vi "PH_PPPA_PowerUnit.PC PU on.vi"(0 "i ref in":refnum<vi>, 2 "PU on":bool, 5 "error in (no error)":errorcluster) -> (14 "i ref out":refnum<vi>, 19 "error out":errorcluster)   [LabVIEW 2014, in "PH_PPPA_PowerUnit.lvlib"]
doc: "This is the action VI of the PU on event case. Depending on the inout it does the following:\n\nfalse: set save state\ntrue: if the PreAmp is not disabled and State SM = \"Stand by\", a state change request is send to SM to get \"Switch PU on\" and the attribute \"PU in use\" is set to true. \nelse: GUI Knob is resetted"
uses:
  PH_PPPA_PowerUnit.lvlib
  PH_Basics/PH_PowerUnit_BaseClass/PH_PowerUnit_BaseClass.SM States.ctl
  PH_Basics/PH_PowerUnit_BaseClass/PH_PowerUnit_BaseClass.lvlib
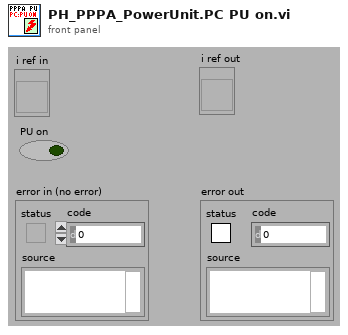
[diagram p1: front panel]
types:
  T1 = typedef "PH_PowerUnit_BaseClass.lvlib/PH_PowerUnit_BaseClass.SM States.ctl" = enum16{".", "Stand by", "Switch PU on", "Configure", "Set Default Voltage", "Set STANDBY", "Set READY", "Wait for Shot Cmd", "Open Dump Rods", "Open Ross Relais", "Close Ross Relais", "Switch PSU on", "Switch PSU off", "Charge", "Switch GD Channel on", "Close Dump Rods", "Rods-TO", "RR-TO", "PSU-TO", "Trigger-TO"}
  T2 = typedef "PH_PPPA_PowerUnit.lvlib/PH_PPPA_PowerUnit.i attribute.ctl" = cluster{"GUI Refs":cluster{"Ignitron":refnum<vi>, "Rossrelais":refnum<vi>, "Set Voltage":refnum<vi>, "PSU":refnum<vi>, "EOC":refnum<vi>, "Trigger":refnum<vi>}, "Ignitron":T3, "PSU":T5, "Dump Ross Relais":T6, "Trigger":cluster{"State Device":T4, "linked?":bool}, "Timing Settings":cluster{"Prdc Fast?":bool, "Default Value Periodic Interval":i32, "Mercury on since":dbl, "Warm up Time Mercury [s]":dbl}, "Set Voltage [V]":dbl, "19er Ignitionbox":string}
  T3 = typedef "PH_PP_Common.lvlib/PH_PP_Common.Ignitron Attributes.ctl" = cluster{"State Device":T4, "linked?":bool}
  T4 = typedef "PH_StatusHandler.lvlib/PH_StatusHandler.Status.ctl" = i16
  T5 = typedef "PH_PP_Common.lvlib/PH_PP_Common.PSU Attributes.ctl" = cluster{"lower limit [V]":dbl, "upper limit [V]":dbl, "Voltage set":bool, "State Device":T4, "linked?":bool}
  T6 = typedef "PH_PP_Common.lvlib/PH_PP_Common.Ross Relais Attributes.ctl" = cluster{"State Device":T4, "linked?":bool}
  T7 = typedef "PH_PowerUnit_BaseClass.lvlib/PH_PowerUnit_BaseClass.i attribute.ctl" = cluster{"Constructor finished":bool, "PU":cluster{"In use":bool, "Service ID in use":i32, "GUI Ref":refnum<vi>}, "Enabling":cluster{"State":T8, "GUI Ref":refnum<vi>}, "Timing":cluster{"Last Shot":dbl, "Time between Shots [Sec]":dbl, "Waiting Time over?":bool, "Service ID Waiting Time":i32, "GUI Ref":refnum<vi>, "Instance":cluster{"Status":T4, "linked?":bool, "GUI Ref":refnum<vi>}}, "Sequencer":cluster{"SM State":string, "GUI Ref":refnum<vi>, "linked":bool}, "Subscribed Trendmssgs":cluster{"Tagname":string, "Status":T4, "linked?":bool, "Shot Condition":T4, "GUI Ref":refnum<vi>}[], "PP PU":T9, "Default Voltage (V)":dbl, "GUI Refs":T10, "PSDB data":cluster{"Shot Voltage [V]":dbl, "State TO SM":T1, "Write 2 early":bool}, "State TO SM":T1}
  T8 = typedef "PH_SystemInformation.lvlib/PH_SystemInformationEnabling State.ctl" = i32
  T9 = typedef "PH_PP_Common.lvlib/PH_PP_Common.PUs.ctl" = enum16{"no Info", "PA-19mm-1", "PA-19mm-2", "PA-45mm-PILC", "PA-45mm-MAIN", "MA-PU-1", "MA-PU-2", "MA-PU-3", "MA-PU-4", "MA-PU-5", "MA-PU-6", "MA-FR", "MA-PILC", "PA-45mm-DP"}
  T10 = typedef "PH_PowerUnit_BaseClass.lvlib/PH_PowerUnit_BaseClass.GUI Refs.ctl" = cluster{"Delete Inst":refnum<vi>, "State TO SM":refnum<vi>, "State SM":refnum<vi>, "Fire":refnum<vi>}
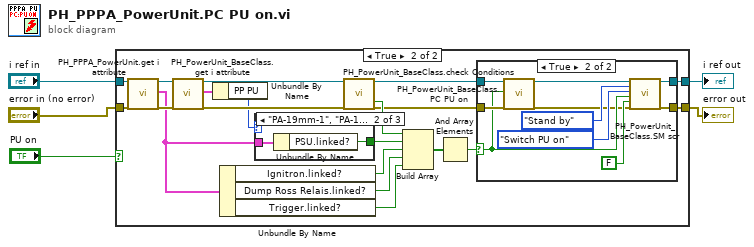
[diagram p0: block diagram]
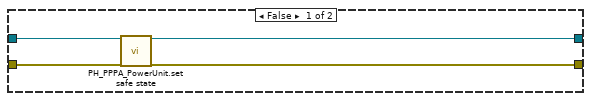
[diagram p2: hidden frame]
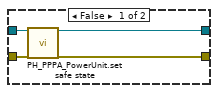
[diagram p3: hidden frame]
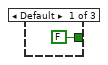
[diagram p4: hidden frame]
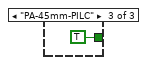
[diagram p5: hidden frame]
diagram:
  n1 = case shown="True" "PU on" {
    tunnel: "i ref in" -> [w9 w24]
    tunnel: [w8 w29] -> w5
    tunnel: "error in (no error)" -> [w7 w23]
    tunnel: [w6 w28] -> w4
    frame False {
      n2 = call "PH_PPPA_PowerUnit.set safe state.vi"("i ref in"=w9, "error in (no error)"=w7) -> ("i ref out"=w8:refnum<vi>, "error out"=w6:errorcluster)  [unwired: 16 in]
    }
    frame True {
      n3 = call "PH_PPPA_PowerUnit.get i attribute.vi"("i ref in"=w24, "error in (no error)"=w23) -> ("i ref out"=w22:refnum<vi>, "i attribute"=w18:T2, "error out"=w21:errorcluster)  [unwired: 15 in]
      n4 = call "PH_PowerUnit_BaseClass.get i attribute.vi"("i ref in"=w22, "error in (no error)"=w21) -> ("i ref out"=w20:refnum<vi>, "i attribute"=w13:T7, "error out"=w19:errorcluster)  [unwired: 15 in]
      n5 = Unbundle By Name(w13) -> ("PP PU"=w12:T9)
      n6 = Unbundle By Name(w18) -> ("Ignitron.linked?"=w17:bool, "Dump Ross Relais.linked?"=w16:bool, "Trigger.linked?"=w15:bool)
      n7 = case shown="\"PA-19mm-1\", \"PA-19mm-2\", \"PA-45mm-MAIN\"" w12 {
        tunnel: w18 -> [_ w46 _]
        tunnel: [FALSE ("linked?") w45 TRUE ("linked?")] -> w25
        frame Default {
        }
        frame "PA-19mm-1", "PA-19mm-2", "PA-45mm-MAIN" {
          n8 = Unbundle By Name(w46) -> ("PSU.linked?"=w45:bool)
        }
        frame "PA-45mm-PILC" {
        }
      }
      n9 = call "PH_PowerUnit_BaseClass.check Conditions.vi"("VI in"=w20, "error in (no error)"=w19) -> ("VI out"=w11:refnum<vi>, "Ready to switch PU on"=w26:bool, "error out"=w10:errorcluster)  [unwired: 14 in, 1 out]
      n10 = Build Array(w26, w25, w17, w16, w15) -> (w27:bool[])
      n11 = And Array Elements(Boolean array=w27) -> (logical AND=w14:bool)
      n12 = case shown="True" w14 {
        selector: w14 -> [_ w37]
        tunnel: w10 -> [w32 w43]
        tunnel: w11 -> [w33 w42]
        tunnel: [w31 w40] -> w29
        tunnel: [w30 w41] -> w28
        frame False {
          n13 = call "PH_PPPA_PowerUnit.set safe state.vi"("i ref in"=w33, "error in (no error)"=w32) -> ("i ref out"=w31:refnum<vi>, "error out"=w30:errorcluster)  [unwired: 16 in]
        }
        frame True {
          n14 = call "PH_PowerUnit_BaseClass.PC PU on.vi"("i ref in"=w42, "PU on"=w37, "error in (no error)"=w43) -> ("i ref out"=w35:refnum<vi>, "error out"=w34:errorcluster)  [unwired: 15 in]
          n15 = call "PH_PowerUnit_BaseClass.SM scr.vi"("VI in"=w35, "Current SM State (condition)"=PH_PowerUnit_BaseClass.SM_States."Stand by", "Wanted SM State"=PH_PowerUnit_BaseClass.SM_States."Switch PU on", "Further change condition"=w37, "PU in use is condition? (true)"=FALSE, "error in (no error)"=w34) -> ("VI out"=w40:refnum<vi>, "error out"=w41:errorcluster)  [unwired: 12 in]
        }
      }
    }
  }
  "error out" <- w4
  "i ref out" <- w5
